vi "RichToFlatcif_manager_PluginStatus.vi"(5 "OutputClusterType":T1, 11 "InputCluster":T16) -> (3 "OutputCluster":T1)   [LabVIEW 2021, in "CIF_Manager_client.lvlib"]
uses:
  CIF_Manager_client.lvlib
  cif_manager_PluginStatus.ctl
  cif_manager_PluginName.ctl
  cif_plugincore_StatusData.ctl
  cif_plugincore_StatusData_PluginState.ctl
  cif_plugincore_TimingStatistics.ctl
  cif_common_TimingStats.ctl
  cif_plugincore_FifoStatistics.ctl
  cif_plugincore_Error.ctl
  cif_plugincore_MonitorDoubles.ctl
  cif_plugincore_MonitorU64.ctl
  cif_plugincore_MonitorI64.ctl
  cif_channelcore_Channels.ctl
  cif_channelcore_Channel.ctl
  cif_channelcore_ChannelDirection.ctl
  cif_channelcore_ChannelPattern.ctl
  cif_manager_PluginStatus_Flat.ctl
  cif_manager_PluginName_Flat.ctl
  cif_plugincore_StatusData_Flat.ctl
  cif_plugincore_TimingStatistics_Flat.ctl
  cif_common_TimingStats_Flat.ctl
  cif_plugincore_FifoStatistics_Flat.ctl
  cif_plugincore_Error_Flat.ctl
  cif_plugincore_MonitorDoubles_Flat.ctl
  cif_plugincore_MonitorU64_Flat.ctl
  cif_plugincore_MonitorI64_Flat.ctl
  cif_channelcore_Channels_Flat.ctl
  cif_channelcore_Channel_Flat.ctl
  RichToFlatcif_plugincore_TimingStatistics.vi
  RichToFlatcif_plugincore_FifoStatistics.vi
  RichToFlatcif_plugincore_Error.vi
  RichToFlatcif_plugincore_MonitorDoubles.vi
  RichToFlatcif_plugincore_MonitorU64.vi
  RichToFlatcif_plugincore_MonitorI64.vi
  RichToFlatcif_channelcore_Channel.vi
  RichToFlatcif_common_TimingStats.vi
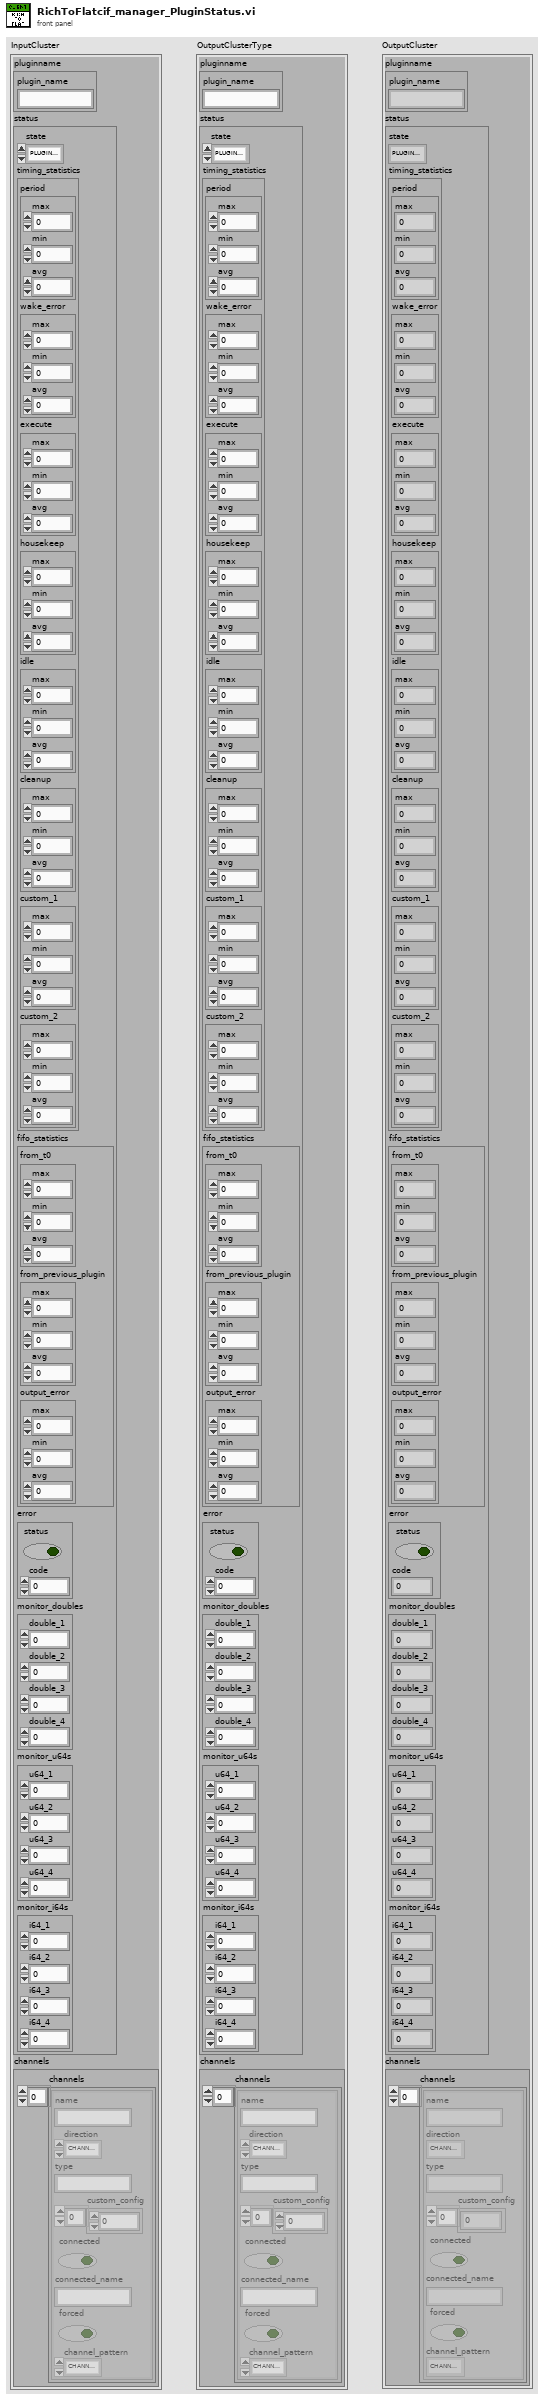
[diagram p1: front panel]
types:
  T1 = typedef "CIF_Manager_client.lvlib/cif_manager_PluginStatus_Flat.ctl" = cluster{"pluginname":T2, "status":T3, "channels":T12}
  T2 = typedef "CIF_Manager_client.lvlib/cif_manager_PluginName_Flat.ctl" = cluster{"plugin_name":string}
  T3 = typedef "CIF_Manager_client.lvlib/cif_plugincore_StatusData_Flat.ctl" = cluster{"state":T4, "timing_statistics":T5, "fifo_statistics":T7, "error":T8, "monitor_doubles":T9, "monitor_u64s":T10, "monitor_i64s":T11}
  T4 = typedef "CIF_Manager_client.lvlib/cif_plugincore_StatusData_PluginState.ctl" = enum32{"PLUGINSTATE_UNKNOWN", "PLUGINSTATE_CREATING", "PLUGINSTATE_LISTENING", "PLUGINSTATE_RUNNING", "PLUGINSTATE_CLEANINGUP", "PLUGINSTATE_DESTROYING"}
  T5 = typedef "CIF_Manager_client.lvlib/cif_plugincore_TimingStatistics_Flat.ctl" = cluster{"period":T6, "wake_error":T6, "execute":T6, "housekeep":T6, "idle":T6, "cleanup":T6, "custom_1":T6, "custom_2":T6}
  T6 = typedef "CIF_Manager_client.lvlib/cif_common_TimingStats_Flat.ctl" = cluster{"max":i64, "min":i64, "avg":dbl}
  T7 = typedef "CIF_Manager_client.lvlib/cif_plugincore_FifoStatistics_Flat.ctl" = cluster{"from_t0":T6, "from_previous_plugin":T6, "output_error":T6}
  T8 = typedef "CIF_Manager_client.lvlib/cif_plugincore_Error_Flat.ctl" = cluster{"status":bool, "code":i32}
  T9 = typedef "CIF_Manager_client.lvlib/cif_plugincore_MonitorDoubles_Flat.ctl" = cluster{"double_1":dbl, "double_2":dbl, "double_3":dbl, "double_4":dbl}
  T10 = typedef "CIF_Manager_client.lvlib/cif_plugincore_MonitorU64_Flat.ctl" = cluster{"u64_1":u64, "u64_2":u64, "u64_3":u64, "u64_4":u64}
  T11 = typedef "CIF_Manager_client.lvlib/cif_plugincore_MonitorI64_Flat.ctl" = cluster{"i64_1":i64, "i64_2":i64, "i64_3":i64, "i64_4":i64}
  T12 = typedef "CIF_Manager_client.lvlib/cif_channelcore_Channels_Flat.ctl" = cluster{"channels":T13[]}
  T13 = typedef "CIF_Manager_client.lvlib/cif_channelcore_Channel_Flat.ctl" = cluster{"name":string, "direction":T14, "type":string, "custom_config":u8[], "connected":bool, "connected_name":string, "forced":bool, "channel_pattern":T15}
  T14 = typedef "CIF_Manager_client.lvlib/cif_channelcore_ChannelDirection.ctl" = enum32{"CHANNELDIRECTION_UNKNOWN", "CHANNELDIRECTION_PUBLISHER", "CHANNELDIRECTION_SUBSCRIBER"}
  T15 = typedef "CIF_Manager_client.lvlib/cif_channelcore_ChannelPattern.ctl" = enum32{"CHANNELPATTERN_UNKNOWN", "CHANNELPATTERN_TAG", "CHANNELPATTERN_FIFO", "CHANNELPATTERN_MULTIFIFO", "CHANNELPATTERN_BACKPRESSUREFIFO"}
  T16 = typedef "CIF_Manager_client.lvlib/cif_manager_PluginStatus.ctl" = cluster{"pluginname":T17, "status":T18, "channels":T26}
  T17 = typedef "CIF_Manager_client.lvlib/cif_manager_PluginName.ctl" = cluster{"plugin_name":string}
  T18 = typedef "CIF_Manager_client.lvlib/cif_plugincore_StatusData.ctl" = cluster{"state":T4, "timing_statistics":T19, "fifo_statistics":T21, "error":T22, "monitor_doubles":T23, "monitor_u64s":T24, "monitor_i64s":T25}
  T19 = typedef "CIF_Manager_client.lvlib/cif_plugincore_TimingStatistics.ctl" = cluster{"period":T20, "wake_error":T20, "execute":T20, "housekeep":T20, "idle":T20, "cleanup":T20, "custom_1":T20, "custom_2":T20}
  T20 = typedef "CIF_Manager_client.lvlib/cif_common_TimingStats.ctl" = cluster{"max":i64, "min":i64, "avg":dbl}
  T21 = typedef "CIF_Manager_client.lvlib/cif_plugincore_FifoStatistics.ctl" = cluster{"from_t0":T20, "from_previous_plugin":T20, "output_error":T20}
  T22 = typedef "CIF_Manager_client.lvlib/cif_plugincore_Error.ctl" = cluster{"status":bool, "code":i32}
  T23 = typedef "CIF_Manager_client.lvlib/cif_plugincore_MonitorDoubles.ctl" = cluster{"double_1":dbl, "double_2":dbl, "double_3":dbl, "double_4":dbl}
  T24 = typedef "CIF_Manager_client.lvlib/cif_plugincore_MonitorU64.ctl" = cluster{"u64_1":u64, "u64_2":u64, "u64_3":u64, "u64_4":u64}
  T25 = typedef "CIF_Manager_client.lvlib/cif_plugincore_MonitorI64.ctl" = cluster{"i64_1":i64, "i64_2":i64, "i64_3":i64, "i64_4":i64}
  T26 = typedef "CIF_Manager_client.lvlib/cif_channelcore_Channels.ctl" = cluster{"channels":T27[]}
  T27 = typedef "CIF_Manager_client.lvlib/cif_channelcore_Channel.ctl" = cluster{"name":string, "direction":T14, "type":string, "custom_config":u8[], "connected":bool, "connected_name":string, "forced":bool, "channel_pattern":T15}
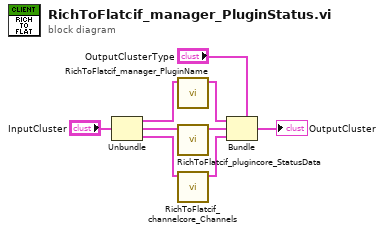
[diagram p0: block diagram]
diagram:
  n1 = Unbundle "Unbundle"("InputCluster") -> ("pluginname"=w6:T17, "status"=w4:T18, "channels"=w2:T26)
  n2 = call "RichToFlatcif_manager_PluginName.vi"("InputCluster"=w6) -> ("OutputCluster"=w5:T2)  [unwired: 10 in]
  n3 = call "RichToFlatcif_plugincore_StatusData.vi"("InputCluster"=w4) -> ("OutputCluster"=w3:T3)  [unwired: 10 in]
  n4 = call "RichToFlatcif_channelcore_Channels.vi"("InputCluster"=w2) -> ("OutputCluster"=w1:T12)  [unwired: 10 in]
  n5 = Bundle "Bundle"(cluster="OutputClusterType", "pluginname"=w5, "status"=w3, "channels"=w1) -> (→"OutputCluster":T1)
